vi "abs_pressure.vi"(0 "Input Voltage":dynamicdata(graph), 1 "Offset[Pa]":dbl) -> (2 "Absolute Pressure":dbl, 3 "Adj Absolute Pressure":dbl, 4 "Adj Absolute Pressure Array":dynamicdata(graph))   [LabVIEW 2016]
uses:
  <vilib>/express/express arith-compare/Formula/XNode/ExpressFormulaBlockNode.xnode
  <vilib>/express/express shared/transition.llb/Dynamic To Waveform Array.vi
  <vilib>/express/express arith-compare/Formula/Block/exnFormulaBlock how many pts in the wave.vi
  <vilib>/express/express shared/ex_Modify Signal Name.vi
  <vilib>/express/express shared/transition.llb/Waveform Array To Dynamic.vi
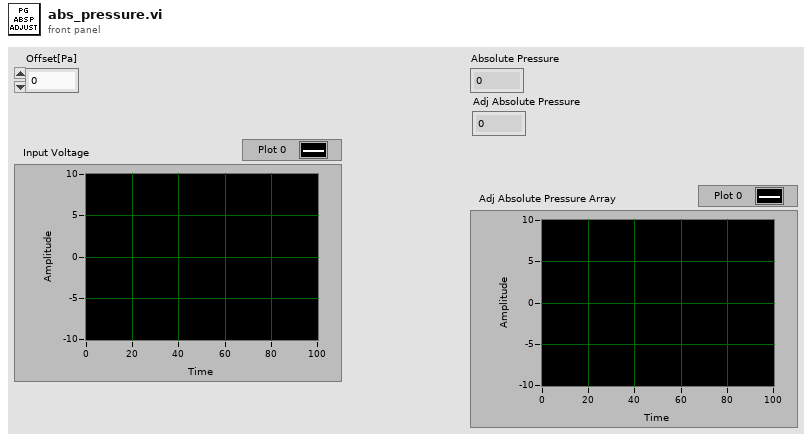
[diagram p1: front panel]
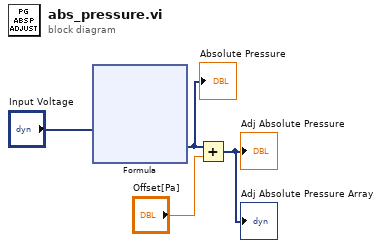
[diagram p0: block diagram]
diagram:
  n1 = xnode "Formula"("V"="Input Voltage") -> ("Result"=w4:dynamicdata)  [unwired: 1 in, 1 out]
  "Absolute Pressure" <- w4
  n2 = Add(x=w4, y="Offset[Pa]") -> (x+y=→"Adj Absolute Pressure" →"Adj Absolute Pressure Array":dynamicdata)
